vi "Database_MLFB_Decoding.vi"(4 "error in":errorcluster, 5 "Language":T2, 6 "MLFB":string, 7 "connection reference":T1) -> (0 "error out":errorcluster, 1 "Message":string, 2 "MLFB_DATA":T3, 3 "connection reference out":T1)   [LabVIEW 2015]
uses:
  CustomControl/MLFB Info.ctl
  CustomControl/Lang_Control.ctl
  <vilib>/addons/database/Connection.llb/Conn ObjectReference.ctl
  <vilib>/addons/database/_DB Variant To Data/Database Variant To Data.xnode
  <vilib>/addons/database/NI_Database_API.lvlib
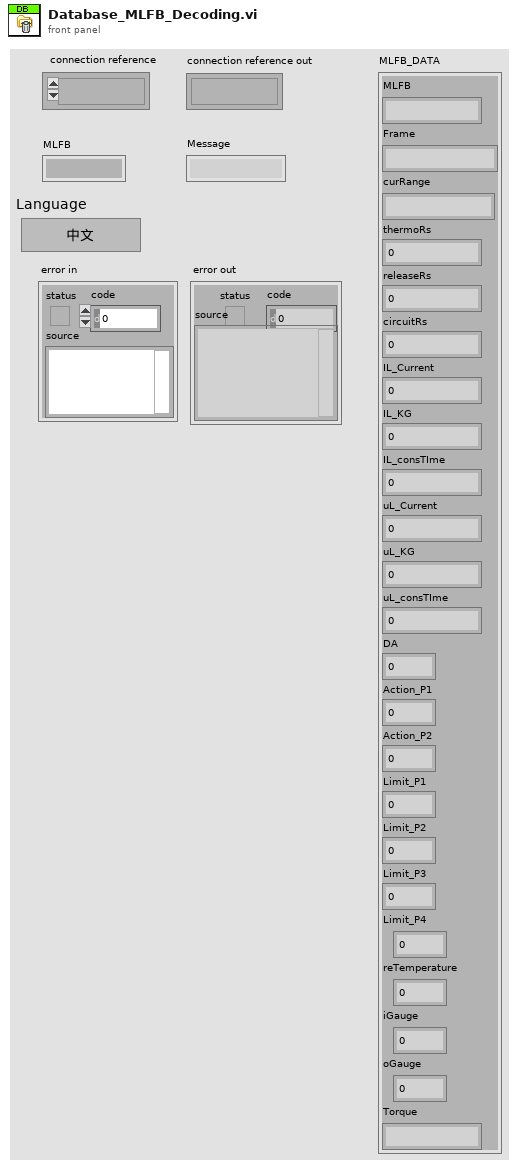
[diagram p1: front panel]
types:
  T1 = typedef "NI_Database_API.lvlib/Conn ObjectReference.ctl" = refnum<k1>
  T2 = typedef "Lang_Control.ctl" = enum16{"中文", "English"}
  T3 = typedef "MLFB Info.ctl" = cluster{"MLFB":string, "Frame":string, "curRange":string, "thermoRs":dbl, "releaseRs":dbl, "circuitRs":dbl, "IL_Current":dbl, "IL_KG":dbl, "IL_consTIme":i32, "uL_Current":dbl, "uL_KG":dbl, "uL_consTIme":i32, "DA":dbl, "Action_P1":i32, "Action_P2":i32, "Limit_P1":i32, "Limit_P2":i32, "Limit_P3":i32, "Limit_P4":i32, "reTemperature":i32, "iGauge":dbl, "oGauge":dbl, "Torque":string}
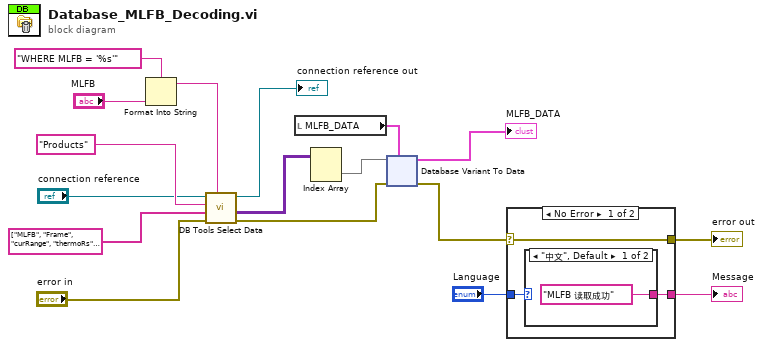
[diagram p0: block diagram]
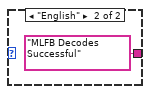
[diagram p2: hidden frame]
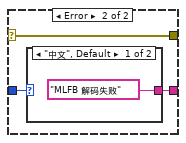
[diagram p3: hidden frame]
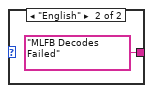
[diagram p4: hidden frame]
diagram:
  n1 = Format Into String(format string="WHERE MLFB = '%s'" ("string"), "MLFB") -> (resulting string=w6:string)  [unwired: 2 in, 1 out]
  n2 = call <vilib>:"DB Tools Select Data.vi"("condition"=w6, "error in (no error)"="error in", "columns"=string[] ["MLFB", "Frame", "curRange", "thermoRs", "releaseRs", "circuitRs", "IL_Current", "IL_KG", "IL_consTime", "uL_Current", "uL_KG", "uL_consTime", "DA", "Release_P1", "Release_P2", "Limit_P1", "Limit_P2", "Limit_P3", "Limit_P4", "reTemperature", "iGauge", "oGauge", "Torque"] ("columns 2"), "table"="Products", "connection reference"="connection reference") -> ("error out"=w11:errorcluster, "data"=w12:variant[][], "connection reference out"=→"connection reference out":T1)  [unwired: 1 in]
  n3 = local read "MLFB_DATA"() -> (w9:T3)
  n4 = Index Array(array=w12) -> (element=w10:variant[])  [unwired: 2 in]
  n5 = xnode "Database Variant To Data"("database variant"=w10, "error in"=w11, "type"=w9) -> ("data"=→"MLFB_DATA":T3, "error out"=w2:errorcluster)
  n6 = case shown="No Error" w2 {
    selector: w2 -> [w20 w25]
    tunnel: [w20 w25] -> w17
    tunnel: "Language" -> [w19 w24]
    tunnel: [w18 w23] -> w13
    frame No Error {
      n7 = case shown="\"中文\", Default" w19 {
        tunnel: ["MLFB 读取成功" "MLFB Decodes Successful"] -> w18
        frame "中文", Default {
        }
        frame "English" {
        }
      }
    }
    frame Error {
      n8 = case shown="\"中文\", Default" w24 {
        tunnel: ["MLFB 解码失败" "MLFB Decodes Failed"] -> w23
        frame "中文", Default {
        }
        frame "English" {
        }
      }
    }
  }
  "error out" <- w17
  "Message" <- w13
